vi "Datasheet Generate.vi"(8 "error in (no error)":errorcluster, 11 "Datasheet Inputs":T1={"Items"=[], "Templates"=[], "Generator Settings"={"Wait? (t)"=TRUE, "ClientPrint? (f)"=FALSE, "Client (\"\")"="", "joinPDF"=FALSE, "Sort Method"=enum."Item", "Export Row (-1=all)"=-1, "Preview"=FALSE, "Estimate Time"=FALSE, "username"="", "jobid"=""}, "Response Queue Name"=""}) -> (0 "error out":errorcluster, 3 "Datasheet Outputs":T4)   [LabVIEW 2011]
uses:
  Datasheet Outputs.ctl
  Datasheet Report Info.ctl
  Datasheet Inputs.ctl
  www/cgi-bin/_cgi-lib/TDM_INDEX Record.ctl
  Datasheet Generator Settings.ctl
  lib/datasheet script data.ctl
  Addons/internet/utils/keyedarr.llb/Keyed Array.ctl
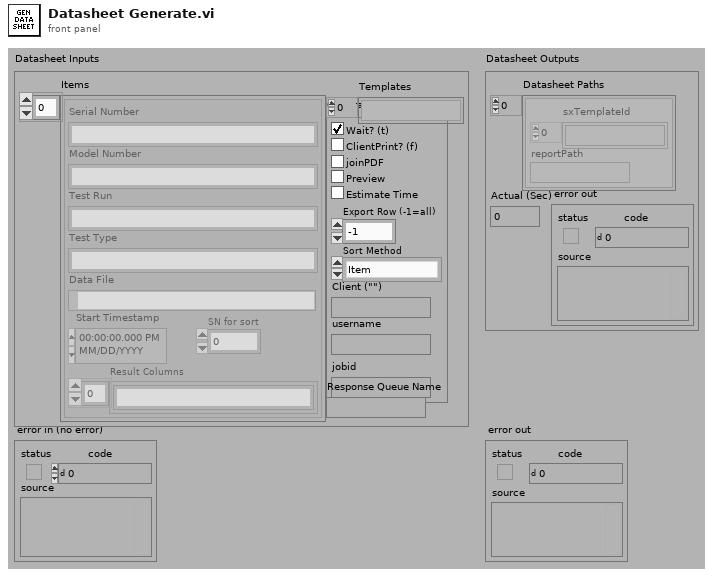
[diagram p1: front panel]
types:
  T1 = typedef "DATASHEET INPUTS.ctl" = cluster{"Items":T2[], "Templates":string[], "Generator Settings":T3, "Response Queue Name":string}
  T2 = typedef "TDM_INDEX Record.ctl" = cluster{"Model Number":string, "SN for sort":i32, "Test Type":string, "Test Run":string, "Serial Number":string, "Start Timestamp":timestamp, "Data File":path, "Result Columns":string[]}
  T3 = typedef "DATASHEET Generator Settings.ctl" = cluster{"Wait? (t)":bool, "ClientPrint? (f)":bool, "Client (\"\")":string, "joinPDF":bool, "Sort Method":enum16{"Item", "Template", "No Sort"}, "Export Row (-1=all)":i32, "Preview":bool, "Estimate Time":bool, "username":string, "jobid":string}
  T4 = typedef "Datasheet Outputs.ctl" = cluster{"Datasheet Paths":T5[], "Actual (Sec)":i32, "error out":errorcluster}
  T5 = typedef "Datasheet Report Info.ctl" = cluster{"sxTemplateId":string[], "reportPath":path}
  T6 = typedef "datasheet script data.ctl" = cluster{"Script":path, "Parameters":T7, "sxTemplateId":string, "Estimate":i32}
  T7 = typedef "Keyed Array.ctl" = cluster{"keys":string[], "values":string[]}
  T8 = typedef "Connection Refnum.ctl" = cluster{"Environment Handle":i32, "Connection Handle":i32}
  T9 = typedef "Template Record.ctl" = cluster{"ixTemplate":i32, "sxTemplateId":string, "sDescription":string, "sCreator":string, "tCreationDate":timestamp, "sModifier":string, "tModifiedDate":timestamp, "sType":string, "sStyle":string, "sFormat":string, "dWidth":dbl, "dHeight":dbl, "sFilename":string, "sScript":string, "sLayout":string, "sEditor":string, "sStyleProcess":string}
  T10 = cluster{"updated Template Record":T9, "Parameters":T7, "estimate to complete (secs)":i32}
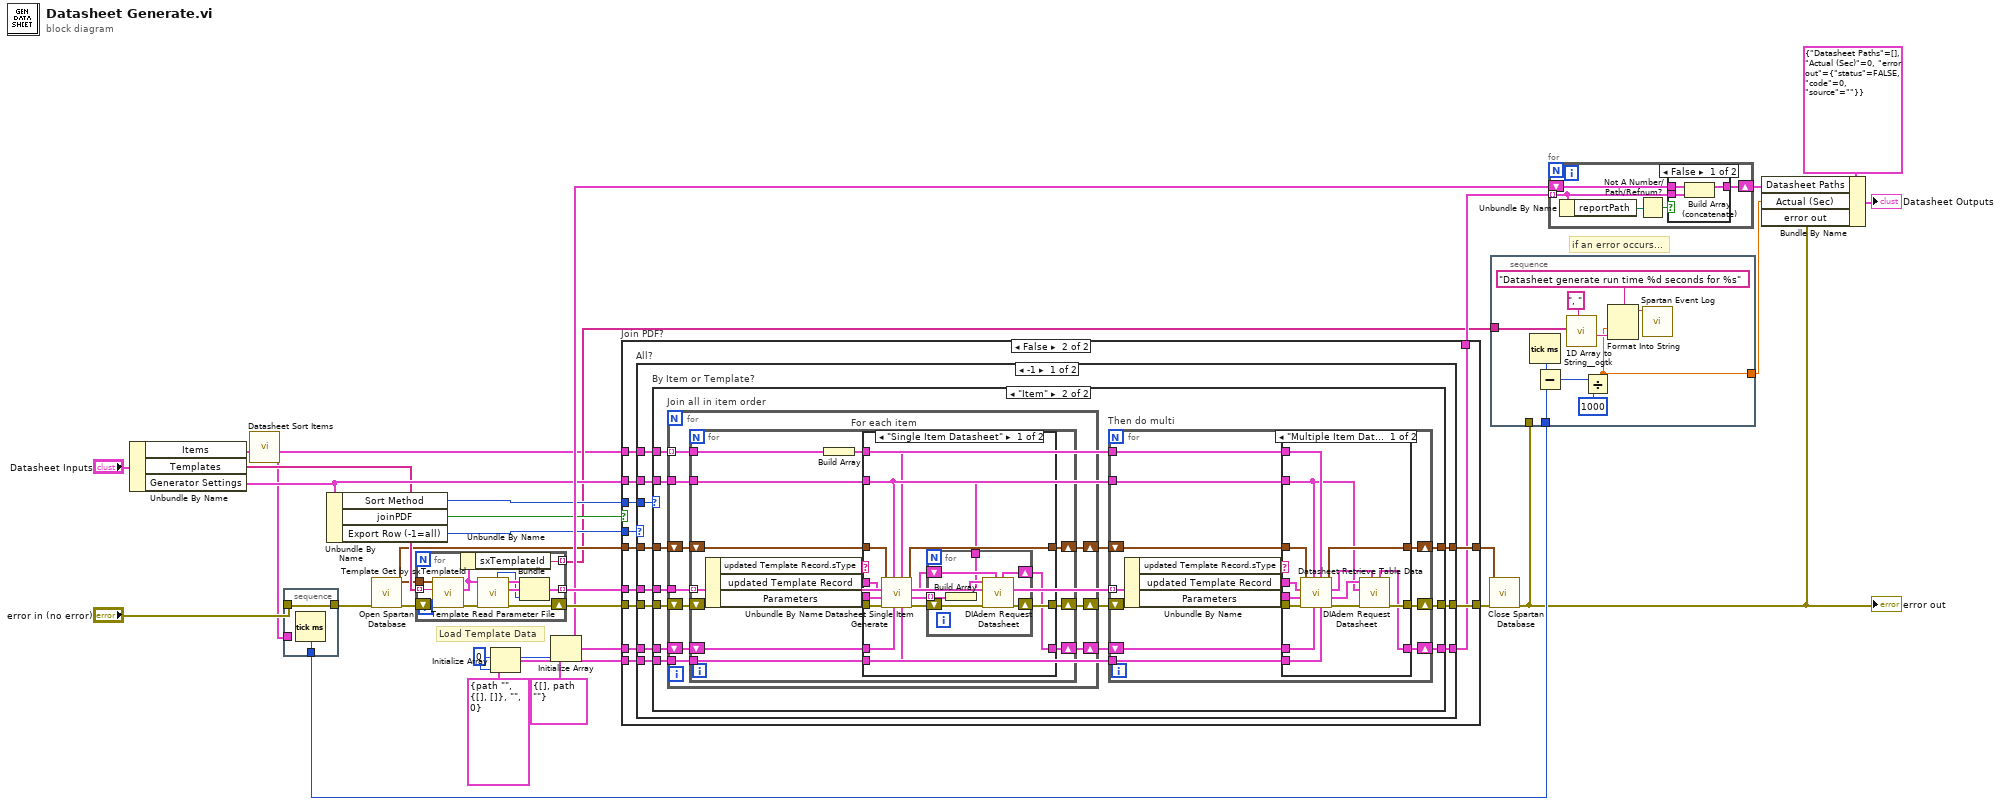
[diagram p0: block diagram]
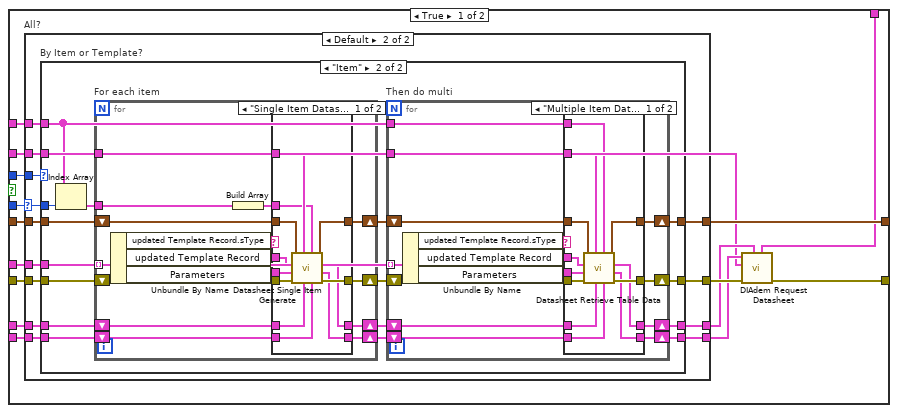
[diagram p2: hidden frame]
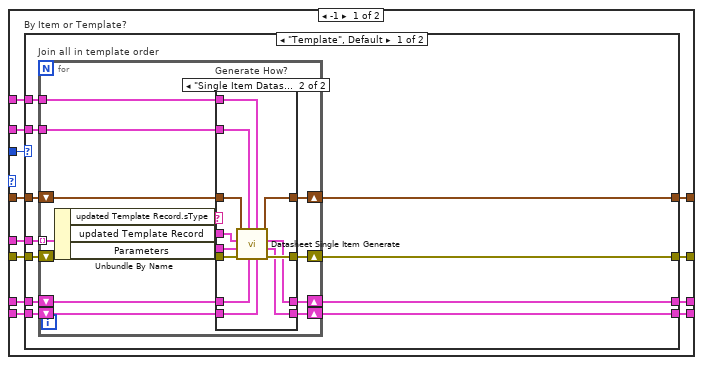
[diagram p3: hidden frame]
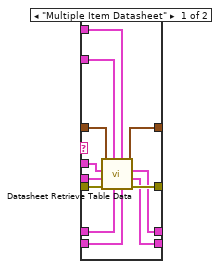
[diagram p4: hidden frame]
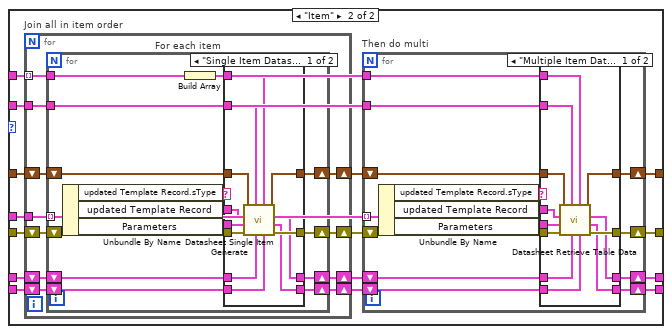
[diagram p5: hidden frame]
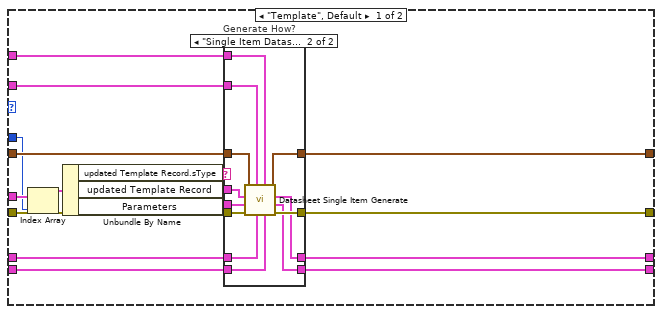
[diagram p8: hidden frame]
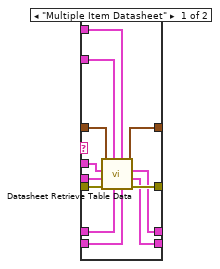
[diagram p9: hidden frame]
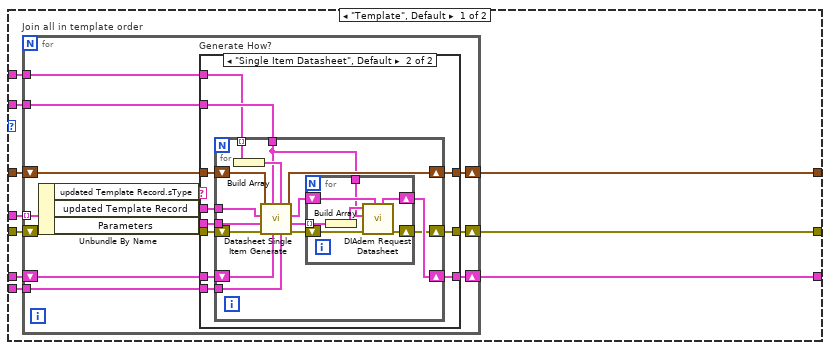
[diagram p12: hidden frame]
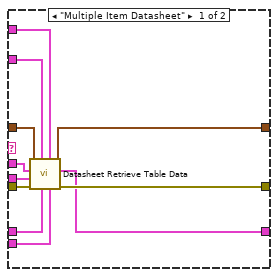
[diagram p13: hidden frame]
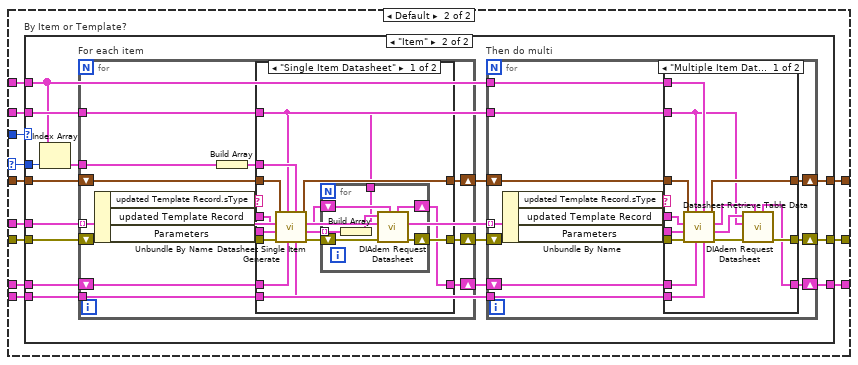
[diagram p16: hidden frame]
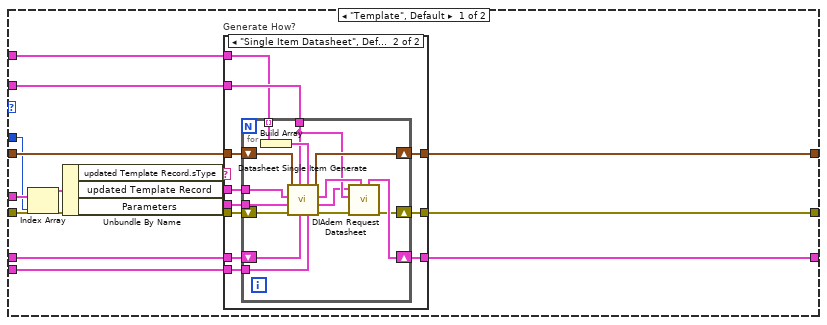
[diagram p17: hidden frame]
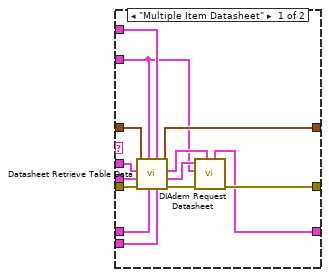
[diagram p18: hidden frame]
diagram:
  w6 = 0 ("dimension size")
  # "if an error occurs..."
  # "Load Template Data"
  n1 = Unbundle By Name("Datasheet Inputs") -> ("Items"=w13:T2[], "Templates"=w12:string[], "Generator Settings"=w14:T3)
  n2 = call "Datasheet Sort Items.vi"("Items"=w13) -> ("Each item tests - Grouped Results"=w1:cluster{"Result Group":T2[]}[])  [unwired: 10 out]
  n3 = stacked-sequence {
    tunnel: [w30] -> w26
    tunnel: [w31] -> w16
    tunnel: "error in (no error)" -> [w30]
    tunnel: w1 -> [_]
    frame #0 {
      n4 = Tick Count (ms)() -> (millisecond timer value=w31:u32)
    }
  }
  n5 = Unbundle By Name(w14) -> ("Sort Method"=w19:enum16{"Item", "Template", "No Sort"}, "joinPDF"=w17:bool, "Export Row (-1=all)"=w18:i32)
  n6 = call "Open Spartan Database.vi"("error in (no error)"=w26) -> ("error out"=w24:errorcluster, "Connection Refnum"=w4:T8)  [unwired: 9 in]
  n7 = for {
    tunnel: w12 -> [w41] mode=indexing
    tunnel: [w37] -> w22 mode=indexing
    shift-right: [w36] -> w23
    shift-left: w24 -> [w40]
    tunnel: w4 -> [w32]
    tunnel: [w34] -> w2 mode=indexing
    n8 = call "Template Get by sxTemplateId.vi"("error in (no error)"=w40, "sxTemplateId (\"\")"=w41, "Connection Refnum"=w32) -> ("error out"=w42:errorcluster, "Template Record"=w35:T9)  [unwired: 7 out]
    n9 = Unbundle By Name(w35) -> ("sxTemplateId"=w34:string)
    n10 = call "Template Read Parameter File.vi"("error in (no error)"=w42, "Template Record"=w35) -> ("error out"=w36:errorcluster, "Parameters"=w38:T7, "updated Template Record"=w39:T9, "estimate to complete (secs)"=w33:i32)  [unwired: 1 in, 5 out]
    n11 = Bundle("updated Template Record"=w39, "Parameters"=w38, "estimate to complete (secs)"=w33) -> (w37:T10)  [unwired: 1 out]
  }
  n12 = Initialize Array(T6 {"Script"=path "", "Parameters"={"keys"=[], "values"=[]}, "sxTemplateId"="", "Estimate"=0} ("Datasheet"), w6) -> (w28:T6[])
  n13 = Initialize Array(T5 {"sxTemplateId"=[], "reportPath"=path ""}, w6) -> (w20:T5[])
  n14 = case "Join PDF?" shown="False" w17 {
    tunnel: w20 -> [w53 w340]
    tunnel: w28 -> [w56 w339]
    tunnel: w14 -> [w43 w346]
    tunnel: [w46 w336] -> w21
    tunnel: w23 -> [w55 w341]
    tunnel: [w47 w337] -> w25
    tunnel: w4 -> [w54 w344]
    tunnel: w1 -> [w52 w347]
    tunnel: w22 -> [w51 w342]
    tunnel: w19 -> [w50 w345]
    tunnel: w18 -> [w49 w343]
    tunnel: [w48 w338] -> w5
    frame True {
      n15 = case "All?" shown="Default" w49 {
        selector: w49 -> [_ w209]
        tunnel: w56 -> [w68 w217]
        tunnel: w43 -> [w60 w213]
        tunnel: [w59 w206] -> w45
        tunnel: w55 -> [w67 w215]
        tunnel: [w57 w207] -> w47
        tunnel: w54 -> [w66 w214]
        tunnel: w53 -> [w65 w216]
        tunnel: w52 -> [w64 w212]
        tunnel: w51 -> [w63 w210]
        tunnel: w50 -> [w62 w211]
        tunnel: [w61 w208] -> w48
        tunnel: [w58 w205] -> w44
        frame -1 {
          n16 = case "By Item or Template?" shown="\"Template\", Default" w62 {
            tunnel: w65 -> [w79 w132]
            tunnel: w68 -> [w78 w131]
            tunnel: [w77 w119] -> w58
            tunnel: w60 -> [w76 w128]
            tunnel: [w75 w120] -> w59
            tunnel: [w74 w121] -> w57
            tunnel: w67 -> [w73 w130]
            tunnel: w66 -> [w72 w129]
            tunnel: w64 -> [w71 w127]
            tunnel: w63 -> [w70 w126]
            tunnel: [w69 w118] -> w61
            frame "Template", Default {
              n17 = for "Join all in template order" {
                tunnel: w76 -> [w93]
                shift-right: [w88] -> w74
                shift-left: w73 -> [w85]
                shift-right: [w83] -> w75
                shift-left: w79 -> [w84]
                tunnel: w71 -> [w92]
                shift-right: [w91] -> w77
                shift-left: w78 -> [w90]
                tunnel: w70 -> [w87] mode=indexing
                shift-right: [w80] -> w69
                shift-left: w72 -> [w89]
                n18 = Unbundle By Name(w87) -> ("updated Template Record.sType"=w81:string, "updated Template Record"=w86:T9, "Parameters"=w82:T7)
                n19 = case "Generate How?" shown="\"Single Item Datasheet\", Default" w81 {
                  tunnel: w85 -> [w96 w116]
                  tunnel: [w99 w115] -> w83
                  tunnel: [w105 w117] -> w88
                  tunnel: w93 -> [w103 w109]
                  tunnel: w89 -> [w98 w113]
                  tunnel: w92 -> [w104 w108]
                  tunnel: w86 -> [w95 w112]
                  tunnel: [w100 w114] -> w91
                  tunnel: w90 -> [w101 w110]
                  tunnel: w84 -> [w102 w111]
                  tunnel: w82 -> [w97 w107]
                  tunnel: [w94 w106] -> w80
                  frame "Multiple Item Datasheet" {
                    n20 = call "Datasheet Retrieve Table Data.vi"("Datasheets to Generate"=w101, "Grouped Results"=w104, "Paths"=w102, "Generator Settings"=w103, "error in (no error)"=w96, "Parameters"=w97, "Template Record"=w95, "Connection Refnum"=w98) -> ("error out"=w105:errorcluster, "Datasheets to Generate"=w100:T6[], "Paths"=w99:T5[], "Connection Refnum"=w94:T8)
                  }
                  frame "Single Item Datasheet", Default {
                    n21 = call "Datasheet Single Item Generate.vi"("Datasheets to Generate"=w110, "Grouped Results"=w108, "Paths"=w111, "Generator Settings"=w109, "error in (no error)"=w116, "Parameters"=w107, "Template Record"=w112, "Connection Refnum"=w113) -> ("error out"=w117:errorcluster, "Datasheets Generated"=w114:T6[], "Paths"=w115:T5[], "Connection Refnum"=w106:T8)
                  }
                }
              }
            }
            frame "Item" {
              n22 = for "Join all in item order" {
                tunnel: w128 -> [w170]
                tunnel: w127 -> [w165] mode=indexing
                shift-right: [w169] -> w125
                shift-left: w132 -> [w173]
                shift-right: [w168] -> w123
                shift-left: w130 -> [w167]
                shift-right: [w171] -> w124
                shift-left: w131 -> [w172]
                tunnel: w126 -> [w164]
                shift-right: [w163] -> w122
                shift-left: w129 -> [w166]
                n23 = for "For each item" {
                  tunnel: w170 -> [w188]
                  shift-right: [w185] -> w168
                  shift-left: w167 -> [w176]
                  shift-right: [w180] -> w169
                  shift-left: w173 -> [w184]
                  shift-right: [w181] -> w171
                  shift-left: w172 -> [w187]
                  tunnel: w165 -> [w183]
                  tunnel: w164 -> [w179] mode=indexing
                  shift-right: [w174] -> w163
                  shift-left: w166 -> [w186]
                  n24 = Unbundle By Name(w179) -> ("updated Template Record.sType"=w175:string, "updated Template Record"=w178:T9, "Parameters"=w177:T7)
                  n25 = Build Array(w183) -> (w182:cluster{"Result Group":T2[]}[])
                  n26 = case shown="\"Single Item Datasheet\"" w175 {
                    tunnel: w176 -> [w200 w204]
                    tunnel: [w199 w204] -> w185
                    tunnel: w188 -> [w190 _]
                    tunnel: w186 -> [w198 w201]
                    tunnel: w182 -> [w189 _]
                    tunnel: w178 -> [w193 _]
                    tunnel: w177 -> [w194 _]
                    tunnel: w187 -> [w191 w203]
                    tunnel: w184 -> [w192 w202]
                    tunnel: [w196 w203] -> w181
                    tunnel: [w197 w202] -> w180
                    tunnel: [w195 w201] -> w174
                    frame "Single Item Datasheet" {
                      n27 = call "Datasheet Single Item Generate.vi"("Datasheets to Generate"=w191, "Grouped Results"=w189, "Paths"=w192, "Generator Settings"=w190, "error in (no error)"=w200, "Parameters"=w194, "Template Record"=w193, "Connection Refnum"=w198) -> ("error out"=w199:errorcluster, "Datasheets Generated"=w196:T6[], "Paths"=w197:T5[], "Connection Refnum"=w195:T8)
                    }
                    frame Default {
                    }
                  }
                }
              }
              n28 = for "Then do multi" {
                tunnel: w128 -> [w146]
                shift-right: [w143] -> w121
                shift-left: w123 -> [w136]
                shift-right: [w140] -> w120
                shift-left: w125 -> [w142]
                shift-right: [w141] -> w119
                shift-left: w124 -> [w145]
                tunnel: w127 -> [w133]
                tunnel: w126 -> [w139] mode=indexing
                shift-right: [w134] -> w118
                shift-left: w122 -> [w144]
                n29 = Unbundle By Name(w139) -> ("updated Template Record.sType"=w135:string, "updated Template Record"=w138:T9, "Parameters"=w137:T7)
                n30 = case shown="\"Multiple Item Datasheet\"" w135 {
                  tunnel: w136 -> [w158 w162]
                  tunnel: [w157 w162] -> w143
                  tunnel: w146 -> [w148 _]
                  tunnel: w144 -> [w156 w159]
                  tunnel: w133 -> [w147 _]
                  tunnel: w138 -> [w151 _]
                  tunnel: w137 -> [w152 _]
                  tunnel: w145 -> [w149 w161]
                  tunnel: w142 -> [w150 w160]
                  tunnel: [w154 w161] -> w141
                  tunnel: [w155 w160] -> w140
                  tunnel: [w153 w159] -> w134
                  frame "Multiple Item Datasheet" {
                    n31 = call "Datasheet Retrieve Table Data.vi"("Datasheets to Generate"=w149, "Grouped Results"=w147, "Paths"=w150, "Generator Settings"=w148, "error in (no error)"=w158, "Parameters"=w152, "Template Record"=w151, "Connection Refnum"=w156) -> ("error out"=w157:errorcluster, "Datasheets to Generate"=w154:T6[], "Paths"=w155:T5[], "Connection Refnum"=w153:T8)
                  }
                  frame Default {
                  }
                }
              }
            }
          }
        }
        frame Default {
          n32 = case "By Item or Template?" shown="\"Item\"" w211 {
            tunnel: w216 -> [w233 w274]
            tunnel: w217 -> [w232 w273]
            tunnel: [w231 w262] -> w205
            tunnel: w213 -> [w230 w270]
            tunnel: [w229 w263] -> w206
            tunnel: [w228 w264] -> w207
            tunnel: w215 -> [w227 w272]
            tunnel: w214 -> [w226 w271]
            tunnel: w212 -> [w225 w258]
            tunnel: w210 -> [w219 w269]
            tunnel: [w224 w261] -> w208
            tunnel: w209 -> [w218 w260]
            frame "Template", Default {
              n33 = Index Array(array=w219, index=w218) -> (element=w220:T10)
              n34 = Unbundle By Name(w220) -> ("updated Template Record.sType"=w221:string, "updated Template Record"=w223:T9, "Parameters"=w222:T7)
              n35 = case "Generate How?" shown="\"Single Item Datasheet\", Default" w221 {
                tunnel: w227 -> [w236 w256]
                tunnel: [w239 w255] -> w229
                tunnel: [w245 w257] -> w228
                tunnel: w230 -> [w243 w249]
                tunnel: w226 -> [w238 w253]
                tunnel: w225 -> [w244 w248]
                tunnel: w223 -> [w235 w252]
                tunnel: [w240 w254] -> w231
                tunnel: w232 -> [w241 w250]
                tunnel: w233 -> [w242 w251]
                tunnel: w222 -> [w237 w247]
                tunnel: [w234 w246] -> w224
                frame "Multiple Item Datasheet" {
                  n36 = call "Datasheet Retrieve Table Data.vi"("Datasheets to Generate"=w241, "Grouped Results"=w244, "Paths"=w242, "Generator Settings"=w243, "error in (no error)"=w236, "Parameters"=w237, "Template Record"=w235, "Connection Refnum"=w238) -> ("error out"=w245:errorcluster, "Datasheets to Generate"=w240:T6[], "Paths"=w239:T5[], "Connection Refnum"=w234:T8)
                }
                frame "Single Item Datasheet", Default {
                  n37 = call "Datasheet Single Item Generate.vi"("Datasheets to Generate"=w250, "Grouped Results"=w248, "Paths"=w251, "Generator Settings"=w249, "error in (no error)"=w256, "Parameters"=w247, "Template Record"=w252, "Connection Refnum"=w253) -> ("error out"=w257:errorcluster, "Datasheets Generated"=w254:T6[], "Paths"=w255:T5[], "Connection Refnum"=w246:T8)
                }
              }
            }
            frame "Item" {
              n38 = Index Array(array=w258, index=w260) -> (element=w259:cluster{"Result Group":T2[]})
              n39 = for "For each item" {
                tunnel: w270 -> [w289]
                shift-right: [w286] -> w266
                shift-left: w272 -> [w278]
                shift-right: [w282] -> w268
                shift-left: w274 -> [w285]
                shift-right: [w283] -> w267
                shift-left: w273 -> [w288]
                tunnel: w269 -> [w281] mode=indexing
                shift-right: [w276] -> w265
                shift-left: w271 -> [w287]
                tunnel: w259 -> [w275]
                n40 = Unbundle By Name(w281) -> ("updated Template Record.sType"=w277:string, "updated Template Record"=w280:T9, "Parameters"=w279:T7)
                n41 = Build Array(w275) -> (w284:cluster{"Result Group":T2[]}[])
                n42 = case shown="\"Single Item Datasheet\"" w277 {
                  tunnel: w278 -> [w301 w305]
                  tunnel: [w300 w305] -> w286
                  tunnel: w289 -> [w291 _]
                  tunnel: w287 -> [w299 w302]
                  tunnel: w284 -> [w290 _]
                  tunnel: w280 -> [w294 _]
                  tunnel: w279 -> [w295 _]
                  tunnel: w288 -> [w292 w304]
                  tunnel: w285 -> [w293 w303]
                  tunnel: [w297 w304] -> w283
                  tunnel: [w298 w303] -> w282
                  tunnel: [w296 w302] -> w276
                  frame "Single Item Datasheet" {
                    n43 = call "Datasheet Single Item Generate.vi"("Datasheets to Generate"=w292, "Grouped Results"=w290, "Paths"=w293, "Generator Settings"=w291, "error in (no error)"=w301, "Parameters"=w295, "Template Record"=w294, "Connection Refnum"=w299) -> ("error out"=w300:errorcluster, "Datasheets Generated"=w297:T6[], "Paths"=w298:T5[], "Connection Refnum"=w296:T8)
                  }
                  frame Default {
                  }
                }
              }
              n44 = for "Then do multi" {
                tunnel: w270 -> [w319]
                shift-right: [w316] -> w264
                shift-left: w266 -> [w309]
                shift-right: [w313] -> w263
                shift-left: w268 -> [w315]
                shift-right: [w314] -> w262
                shift-left: w267 -> [w318]
                tunnel: w258 -> [w306]
                tunnel: w269 -> [w312] mode=indexing
                shift-right: [w307] -> w261
                shift-left: w265 -> [w317]
                n45 = Unbundle By Name(w312) -> ("updated Template Record.sType"=w308:string, "updated Template Record"=w311:T9, "Parameters"=w310:T7)
                n46 = case shown="\"Multiple Item Datasheet\"" w308 {
                  tunnel: w309 -> [w331 w335]
                  tunnel: [w330 w335] -> w316
                  tunnel: w319 -> [w321 _]
                  tunnel: w317 -> [w329 w332]
                  tunnel: w306 -> [w320 _]
                  tunnel: w311 -> [w324 _]
                  tunnel: w310 -> [w325 _]
                  tunnel: w318 -> [w322 w334]
                  tunnel: w315 -> [w323 w333]
                  tunnel: [w327 w334] -> w314
                  tunnel: [w328 w333] -> w313
                  tunnel: [w326 w332] -> w307
                  frame "Multiple Item Datasheet" {
                    n47 = call "Datasheet Retrieve Table Data.vi"("Datasheets to Generate"=w322, "Grouped Results"=w320, "Paths"=w323, "Generator Settings"=w321, "error in (no error)"=w331, "Parameters"=w325, "Template Record"=w324, "Connection Refnum"=w329) -> ("error out"=w330:errorcluster, "Datasheets to Generate"=w327:T6[], "Paths"=w328:T5[], "Connection Refnum"=w326:T8)
                  }
                  frame Default {
                  }
                }
              }
            }
          }
        }
      }
      n48 = call "DIAdem Request Datasheet.vi"("Paths"=w45, "error in (no error)"=w47, "Generator Settings"=w43, "Datasheets to Generate"=w44) -> ("Paths"=w46:T5[])  [unwired: 1 in, 6 out]
    }
    frame False {
      n49 = case "All?" shown="-1" w343 {
        selector: w343 -> [_ w520]
        tunnel: w339 -> [w358 w528]
        tunnel: w346 -> [w350 w524]
        tunnel: [w349 w517] -> w336
        tunnel: w341 -> [w357 w526]
        tunnel: [w348 w518] -> w337
        tunnel: w344 -> [w356 w525]
        tunnel: w340 -> [w355 w527]
        tunnel: w347 -> [w354 w523]
        tunnel: w342 -> [w353 w521]
        tunnel: w345 -> [w352 w522]
        tunnel: [w351 w519] -> w338
        frame -1 {
          n50 = case "By Item or Template?" shown="\"Item\"" w352 {
            tunnel: w355 -> [w368 w438]
            tunnel: w358 -> [w359 w426]
            tunnel: w350 -> [w367 w435]
            tunnel: [w366 w428] -> w349
            tunnel: [w365 w429] -> w348
            tunnel: w357 -> [w364 w437]
            tunnel: w356 -> [w363 w436]
            tunnel: w354 -> [w362 w434]
            tunnel: w353 -> [w361 w433]
            tunnel: [w360 w427] -> w351
            frame "Template", Default {
              n51 = for "Join all in template order" {
                tunnel: w367 -> [w381]
                shift-right: [w378] -> w365
                shift-left: w364 -> [w375]
                shift-right: [w373] -> w366
                shift-left: w368 -> [w374]
                tunnel: w362 -> [w380]
                tunnel: w361 -> [w377] mode=indexing
                shift-right: [w370] -> w360
                shift-left: w363 -> [w379]
                tunnel: w359 -> [w369]
                n52 = Unbundle By Name(w377) -> ("updated Template Record.sType"=w371:string, "updated Template Record"=w376:T9, "Parameters"=w372:T7)
                n53 = case "Generate How?" shown="\"Single Item Datasheet\", Default" w371 {
                  tunnel: w375 -> [w384 w402]
                  tunnel: [w387 w401] -> w373
                  tunnel: [w392 w403] -> w378
                  tunnel: w381 -> [w390 w397]
                  tunnel: w379 -> [w386 w400]
                  tunnel: w380 -> [w391 w396]
                  tunnel: w376 -> [w383 w399]
                  tunnel: w369 -> [w388 w393]
                  tunnel: w374 -> [w389 w398]
                  tunnel: w372 -> [w385 w395]
                  tunnel: [w382 w394] -> w370
                  frame "Multiple Item Datasheet" {
                    n54 = call "Datasheet Retrieve Table Data.vi"("Datasheets to Generate"=w388, "Grouped Results"=w391, "Paths"=w389, "Generator Settings"=w390, "error in (no error)"=w384, "Parameters"=w385, "Template Record"=w383, "Connection Refnum"=w386) -> ("error out"=w392:errorcluster, "Paths"=w387:T5[], "Connection Refnum"=w382:T8)  [unwired: 1 out]
                  }
                  frame "Single Item Datasheet", Default {
                    n55 = for {
                      tunnel: w399 -> [w416]
                      tunnel: w397 -> [w405]
                      tunnel: w396 -> [w411] mode=indexing
                      tunnel: w395 -> [w414]
                      shift-right: [w409] -> w401
                      shift-left: w398 -> [w415]
                      shift-right: [w413] -> w394
                      shift-left: w400 -> [w417]
                      shift-right: [w407] -> w403
                      shift-left: w402 -> [w418]
                      tunnel: w393 -> [w404]
                      n56 = Build Array(w411) -> (w412:cluster{"Result Group":T2[]}[])
                      n57 = call "Datasheet Single Item Generate.vi"("Datasheets to Generate"=w404, "Grouped Results"=w412, "Paths"=w415, "Generator Settings"=w405, "error in (no error)"=w418, "Parameters"=w414, "Template Record"=w416, "Connection Refnum"=w417) -> ("error out"=w408:errorcluster, "Datasheets Generated"=w406:T6[], "Paths"=w410:T5[], "Connection Refnum"=w413:T8)
                      n58 = for {
                        shift-right: [w422] -> w409
                        shift-left: w410 -> [w423]
                        shift-right: [w425] -> w407
                        shift-left: w408 -> [w424]
                        tunnel: w406 -> [w421] mode=indexing
                        tunnel: w405 -> [w419]
                        n59 = Build Array(w421) -> (w420:T6[])
                        n60 = call "DIAdem Request Datasheet.vi"("Paths"=w423, "error in (no error)"=w424, "Generator Settings"=w419, "Datasheets to Generate"=w420) -> ("error out"=w425:errorcluster, "Paths"=w422:T5[])  [unwired: 1 in, 5 out]
                      }
                    }
                  }
                }
              }
            }
            frame "Item" {
              n61 = for "Join all in item order" {
                tunnel: w435 -> [w477]
                tunnel: w434 -> [w472] mode=indexing
                shift-right: [w476] -> w432
                shift-left: w438 -> [w478]
                shift-right: [w475] -> w431
                shift-left: w437 -> [w474]
                tunnel: w433 -> [w471]
                shift-right: [w470] -> w430
                shift-left: w436 -> [w473]
                tunnel: w426 -> [w469]
                n62 = for "For each item" {
                  tunnel: w477 -> [w492]
                  shift-right: [w490] -> w475
                  shift-left: w474 -> [w482]
                  shift-right: [w486] -> w476
                  shift-left: w478 -> [w489]
                  tunnel: w472 -> [w488]
                  tunnel: w471 -> [w485] mode=indexing
                  shift-right: [w480] -> w470
                  shift-left: w473 -> [w491]
                  tunnel: w469 -> [w479]
                  n63 = Unbundle By Name(w485) -> ("updated Template Record.sType"=w481:string, "updated Template Record"=w484:T9, "Parameters"=w483:T7)
                  n64 = Build Array(w488) -> (w487:cluster{"Result Group":T2[]}[])
                  n65 = case shown="\"Single Item Datasheet\"" w481 {
                    tunnel: w482 -> [w506 w516]
                    tunnel: [w497 w516] -> w490
                    tunnel: w492 -> [w493 _]
                    tunnel: w491 -> [w505 w514]
                    tunnel: w487 -> [w499 _]
                    tunnel: w484 -> [w502 _]
                    tunnel: w483 -> [w503 _]
                    tunnel: w479 -> [w500 _]
                    tunnel: w489 -> [w501 w515]
                    tunnel: [w495 w515] -> w486
                    tunnel: [w504 w514] -> w480
                    frame "Single Item Datasheet" {
                      n66 = call "Datasheet Single Item Generate.vi"("Datasheets to Generate"=w500, "Grouped Results"=w499, "Paths"=w501, "Generator Settings"=w493, "error in (no error)"=w506, "Parameters"=w503, "Template Record"=w502, "Connection Refnum"=w505) -> ("error out"=w498:errorcluster, "Datasheets Generated"=w494:T6[], "Paths"=w496:T5[], "Connection Refnum"=w504:T8)
                      n67 = for {
                        shift-right: [w510] -> w495
                        shift-left: w496 -> [w511]
                        shift-right: [w513] -> w497
                        shift-left: w498 -> [w512]
                        tunnel: w494 -> [w509] mode=indexing
                        tunnel: w493 -> [w507]
                        n68 = Build Array(w509) -> (w508:T6[])
                        n69 = call "DIAdem Request Datasheet.vi"("Paths"=w511, "error in (no error)"=w512, "Generator Settings"=w507, "Datasheets to Generate"=w508) -> ("error out"=w513:errorcluster, "Paths"=w510:T5[])  [unwired: 1 in, 5 out]
                      }
                    }
                    frame Default {
                    }
                  }
                }
              }
              n70 = for "Then do multi" {
                tunnel: w435 -> [w451]
                shift-right: [w449] -> w429
                shift-left: w431 -> [w443]
                shift-right: [w447] -> w428
                shift-left: w432 -> [w448]
                tunnel: w434 -> [w440]
                tunnel: w433 -> [w446] mode=indexing
                shift-right: [w441] -> w427
                shift-left: w430 -> [w450]
                tunnel: w426 -> [w439]
                n71 = Unbundle By Name(w446) -> ("updated Template Record.sType"=w442:string, "updated Template Record"=w445:T9, "Parameters"=w444:T7)
                n72 = case shown="\"Multiple Item Datasheet\"" w442 {
                  tunnel: w443 -> [w465 w468]
                  tunnel: [w456 w468] -> w449
                  tunnel: w451 -> [w454 _]
                  tunnel: w450 -> [w464 w466]
                  tunnel: w440 -> [w458 _]
                  tunnel: w445 -> [w461 _]
                  tunnel: w444 -> [w462 _]
                  tunnel: w439 -> [w459 _]
                  tunnel: w448 -> [w460 w467]
                  tunnel: [w452 w467] -> w447
                  tunnel: [w463 w466] -> w441
                  frame "Multiple Item Datasheet" {
                    n73 = call "Datasheet Retrieve Table Data.vi"("Datasheets to Generate"=w459, "Grouped Results"=w458, "Paths"=w460, "Generator Settings"=w454, "error in (no error)"=w465, "Parameters"=w462, "Template Record"=w461, "Connection Refnum"=w464) -> ("error out"=w457:errorcluster, "Datasheets to Generate"=w455:T6[], "Paths"=w453:T5[], "Connection Refnum"=w463:T8)
                    n74 = call "DIAdem Request Datasheet.vi"("Paths"=w453, "error in (no error)"=w457, "Generator Settings"=w454, "Datasheets to Generate"=w455) -> ("error out"=w456:errorcluster, "Paths"=w452:T5[])  [unwired: 1 in, 5 out]
                  }
                  frame Default {
                  }
                }
              }
            }
          }
        }
        frame Default {
          n75 = case "By Item or Template?" shown="\"Item\"" w522 {
            tunnel: w527 -> [w543 w598]
            tunnel: w528 -> [w542 w584]
            tunnel: w524 -> [w541 w595]
            tunnel: [w540 w589] -> w517
            tunnel: [w539 w590] -> w518
            tunnel: w526 -> [w538 w597]
            tunnel: w525 -> [w537 w596]
            tunnel: w523 -> [w536 w585]
            tunnel: w521 -> [w530 w594]
            tunnel: [w535 w588] -> w519
            tunnel: w520 -> [w529 w587]
            frame "Template", Default {
              n76 = Index Array(array=w530, index=w529) -> (element=w531:T10)
              n77 = Unbundle By Name(w531) -> ("updated Template Record.sType"=w532:string, "updated Template Record"=w534:T9, "Parameters"=w533:T7)
              n78 = case "Generate How?" shown="\"Single Item Datasheet\", Default" w532 {
                tunnel: w538 -> [w552 w563]
                tunnel: [w546 w560] -> w540
                tunnel: [w548 w566] -> w539
                tunnel: w541 -> [w544 w559]
                tunnel: w537 -> [w554 w568]
                tunnel: w536 -> [w557 w558]
                tunnel: w534 -> [w551 w565]
                tunnel: w542 -> [w555 w561]
                tunnel: w543 -> [w556 w562]
                tunnel: w533 -> [w553 w564]
                tunnel: [w550 w567] -> w535
                frame "Multiple Item Datasheet" {
                  n79 = call "Datasheet Retrieve Table Data.vi"("Datasheets to Generate"=w555, "Grouped Results"=w557, "Paths"=w556, "Generator Settings"=w544, "error in (no error)"=w552, "Parameters"=w553, "Template Record"=w551, "Connection Refnum"=w554) -> ("error out"=w549:errorcluster, "Datasheets to Generate"=w545:T6[], "Paths"=w547:T5[], "Connection Refnum"=w550:T8)
                  n80 = call "DIAdem Request Datasheet.vi"("Paths"=w547, "error in (no error)"=w549, "Generator Settings"=w544, "Datasheets to Generate"=w545) -> ("error out"=w548:errorcluster, "Paths"=w546:T5[])  [unwired: 1 in, 5 out]
                }
                frame "Single Item Datasheet", Default {
                  n81 = for {
                    tunnel: w565 -> [w581]
                    tunnel: w559 -> [w571]
                    tunnel: w558 -> [w576] mode=indexing
                    tunnel: w564 -> [w579]
                    shift-right: [w574] -> w560
                    shift-left: w562 -> [w580]
                    shift-right: [w578] -> w567
                    shift-left: w568 -> [w582]
                    shift-right: [w572] -> w566
                    shift-left: w563 -> [w583]
                    tunnel: w561 -> [w570]
                    n82 = Build Array(w576) -> (w577:cluster{"Result Group":T2[]}[])
                    n83 = call "Datasheet Single Item Generate.vi"("Datasheets to Generate"=w570, "Grouped Results"=w577, "Paths"=w580, "Generator Settings"=w571, "error in (no error)"=w583, "Parameters"=w579, "Template Record"=w581, "Connection Refnum"=w582) -> ("error out"=w573:errorcluster, "Datasheets Generated"=w569:T6[], "Paths"=w575:T5[], "Connection Refnum"=w578:T8)
                    n84 = call "DIAdem Request Datasheet.vi"("Paths"=w575, "error in (no error)"=w573, "Generator Settings"=w571, "Datasheets to Generate"=w569) -> ("error out"=w572:errorcluster, "Paths"=w574:T5[])  [unwired: 1 in, 5 out]
                  }
                }
              }
            }
            frame "Item" {
              n85 = Index Array(array=w585, index=w587) -> (element=w586:cluster{"Result Group":T2[]})
              n86 = for "For each item" {
                tunnel: w595 -> [w612]
                shift-right: [w609] -> w592
                shift-left: w597 -> [w602]
                shift-right: [w606] -> w593
                shift-left: w598 -> [w608]
                tunnel: w594 -> [w605] mode=indexing
                shift-right: [w600] -> w591
                shift-left: w596 -> [w610]
                tunnel: w586 -> [w599]
                tunnel: w584 -> [w611]
                n87 = Unbundle By Name(w605) -> ("updated Template Record.sType"=w601:string, "updated Template Record"=w604:T9, "Parameters"=w603:T7)
                n88 = Build Array(w599) -> (w607:cluster{"Result Group":T2[]}[])
                n89 = case shown="\"Single Item Datasheet\"" w601 {
                  tunnel: w602 -> [w626 w636]
                  tunnel: [w617 w636] -> w609
                  tunnel: w612 -> [w616 _]
                  tunnel: w610 -> [w625 w634]
                  tunnel: w607 -> [w619 _]
                  tunnel: w604 -> [w622 _]
                  tunnel: w603 -> [w623 _]
                  tunnel: w611 -> [w620 _]
                  tunnel: w608 -> [w621 w635]
                  tunnel: [w613 w635] -> w606
                  tunnel: [w624 w634] -> w600
                  frame "Single Item Datasheet" {
                    n90 = call "Datasheet Single Item Generate.vi"("Datasheets to Generate"=w620, "Grouped Results"=w619, "Paths"=w621, "Generator Settings"=w616, "error in (no error)"=w626, "Parameters"=w623, "Template Record"=w622, "Connection Refnum"=w625) -> ("error out"=w618:errorcluster, "Datasheets Generated"=w615:T6[], "Paths"=w614:T5[], "Connection Refnum"=w624:T8)
                    n91 = for {
                      shift-right: [w630] -> w613
                      shift-left: w614 -> [w631]
                      shift-right: [w633] -> w617
                      shift-left: w618 -> [w632]
                      tunnel: w615 -> [w629] mode=indexing
                      tunnel: w616 -> [w627]
                      n92 = Build Array(w629) -> (w628:T6[])
                      n93 = call "DIAdem Request Datasheet.vi"("Paths"=w631, "error in (no error)"=w632, "Generator Settings"=w627, "Datasheets to Generate"=w628) -> ("error out"=w633:errorcluster, "Paths"=w630:T5[])  [unwired: 1 in, 5 out]
                    }
                  }
                  frame Default {
                  }
                }
              }
              n94 = for "Then do multi" {
                tunnel: w595 -> [w649]
                shift-right: [w646] -> w590
                shift-left: w592 -> [w640]
                shift-right: [w644] -> w589
                shift-left: w593 -> [w645]
                tunnel: w585 -> [w637]
                tunnel: w594 -> [w643] mode=indexing
                shift-right: [w638] -> w588
                shift-left: w591 -> [w647]
                tunnel: w584 -> [w648]
                n95 = Unbundle By Name(w643) -> ("updated Template Record.sType"=w639:string, "updated Template Record"=w642:T9, "Parameters"=w641:T7)
                n96 = case shown="\"Multiple Item Datasheet\"" w639 {
                  tunnel: w640 -> [w663 w666]
                  tunnel: [w654 w666] -> w646
                  tunnel: w649 -> [w650 _]
                  tunnel: w647 -> [w662 w664]
                  tunnel: w637 -> [w656 _]
                  tunnel: w642 -> [w659 _]
                  tunnel: w641 -> [w660 _]
                  tunnel: w648 -> [w657 _]
                  tunnel: w645 -> [w658 w665]
                  tunnel: [w651 w665] -> w644
                  tunnel: [w661 w664] -> w638
                  frame "Multiple Item Datasheet" {
                    n97 = call "Datasheet Retrieve Table Data.vi"("Datasheets to Generate"=w657, "Grouped Results"=w656, "Paths"=w658, "Generator Settings"=w650, "error in (no error)"=w663, "Parameters"=w660, "Template Record"=w659, "Connection Refnum"=w662) -> ("error out"=w655:errorcluster, "Datasheets to Generate"=w652:T6[], "Paths"=w653:T5[], "Connection Refnum"=w661:T8)
                    n98 = call "DIAdem Request Datasheet.vi"("Paths"=w653, "error in (no error)"=w655, "Generator Settings"=w650, "Datasheets to Generate"=w652) -> ("error out"=w654:errorcluster, "Paths"=w651:T5[])  [unwired: 1 in, 5 out]
                  }
                  frame Default {
                  }
                }
              }
            }
          }
        }
      }
    }
  }
  n99 = call "Close Spartan Database.vi"("error in (no error)"=w25, "Connection Refnum"=w5) -> ("error out"=w3:errorcluster)  [unwired: 9 in]
  "error out" <- w3
  n100 = stacked-sequence {
    tunnel: w16 -> [w675]
    tunnel: w2 -> [w670]
    tunnel: [w667] -> w8
    tunnel: w3 -> [_]
    frame #0 {
      n101 = Tick Count (ms)() -> (millisecond timer value=w676:u32)
      n102 = Subtract(x=w676, y=w675) -> (x-y=w674:u32)
      n103 = call "1D Array to String__ogtk.vi"("delimiter (Tab)"=", ", "Array of Strings"=w670) -> ("delimited string"=w669:string)  [unwired: 9 in]
      n104 = Divide(x=w674, y=u32 1000) -> (x/y=w667:dbl)
      n105 = Format Into String(format string="Datasheet generate run time %d seconds for %s" ("name (unnamed)"), w667, w669) -> (resulting string=w671:string)  [unwired: 2 in, 1 out]
      n106 = call "Spartan Event Log.vi"("message (\"\")"=w671) -> ()  [unwired: 4 in, 4 out]
    }
  }
  n107 = for {
    tunnel: w21 -> [w677] mode=indexing
    shift-right: [w680] -> w10
    shift-left: w20 -> [w681]
    n108 = Unbundle By Name(w677) -> ("reportPath"=w678:path)
    n109 = Not A Number/Path/Refnum?(number/path/refnum=w678) -> (NaN/Path/Refnum?=w679:bool)
    n110 = case shown="False" w679 {
      tunnel: w681 -> [w683 w685]
      tunnel: [w684 w685] -> w680
      tunnel: w677 -> [w682 _]
      frame False {
        n111 = Build Array (concatenate)(w683, w682) -> (w684:T5[])
      }
      frame True {
      }
    }
  }
  n112 = Bundle By Name(cluster=T4 {"Datasheet Paths"=[], "Actual (Sec)"=0, "error out"={"status"=FALSE, "code"=0, "source"=""}} ("OUTPUTS"), "Datasheet Paths"=w10, "Actual (Sec)"=w8, "error out"=w3) -> (→"Datasheet Outputs":T4)
